vi "Write Trace Level.vi"(8 "error in (no error)":errorcluster, 10 "Trace Level":T1(ring)=enum."Error", 11 "System Actor in":refnum<class "System Actor.lvclass">) -> (0 "error out":errorcluster, 3 "System Actor out":refnum<class "System Actor.lvclass">)   [LabVIEW 2014, in "Robot Actor Framework.lvlib" / "System Actor.lvlib" / "System Actor.lvclass"]
uses:
  System Actor.lvclass
  System Actor.lvclass/System Actor.ctl
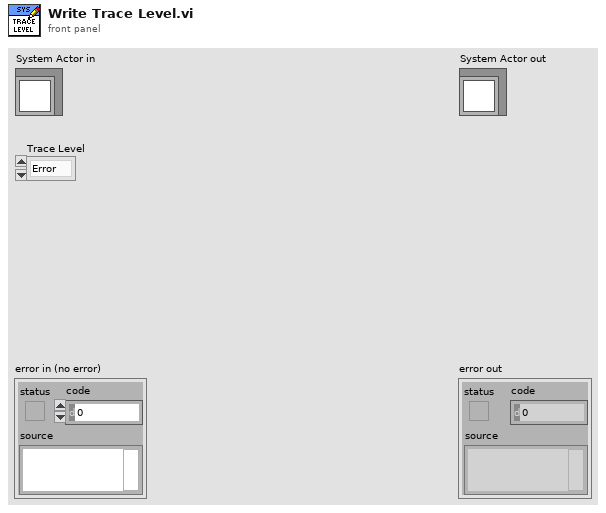
[diagram p1: front panel]
types:
  T1 = enum16{"Critical", "Error", "Warning", "Informational", "Debug"}
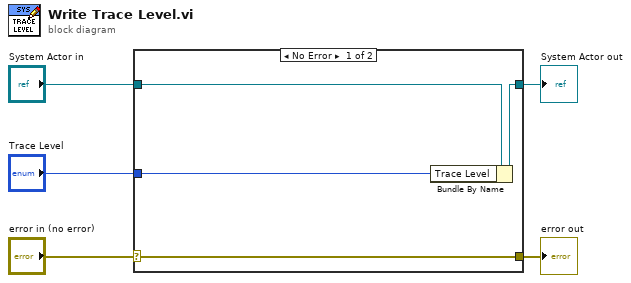
[diagram p0: block diagram]
diagram:
  n1 = case shown="No Error" "error in (no error)" {
    selector: "error in (no error)" -> [w9 w10]
    tunnel: [w9 w10] -> w4
    tunnel: [w7 w11] -> w2
    tunnel: "System Actor in" -> [w8 w11]
    tunnel: "Trace Level" -> [w6 _]
    frame No Error {
      n2 = Bundle By Name(cluster=w8, "Trace Level"=w6) -> (w7:refnum<class "System Actor.lvclass">)
    }
    frame Error {
    }
  }
  "error out" <- w4
  "System Actor out" <- w2
